vi "Sondenmodell.Erdtemperatur.vi"(8 "Error in":errorcluster, 10 "Vorlauftemperatur Solekreislauf [°C]":dbl, 11 "Sondenmodell in":refnum<data-value>) -> (0 "Error out":errorcluster, 3 "Sondenmodell out":refnum<data-value>)   [LabVIEW 2016, in "Sondenmodell.lvclass"]
uses:
  Sondenmodell.lvclass
  Sondenmodell.lvclass/Sondenmodell.ctl
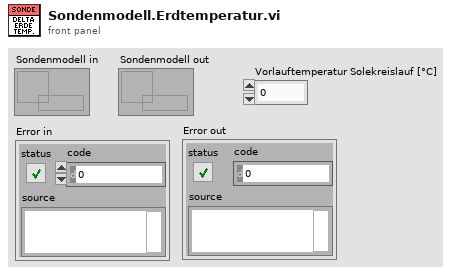
[diagram p1: front panel]
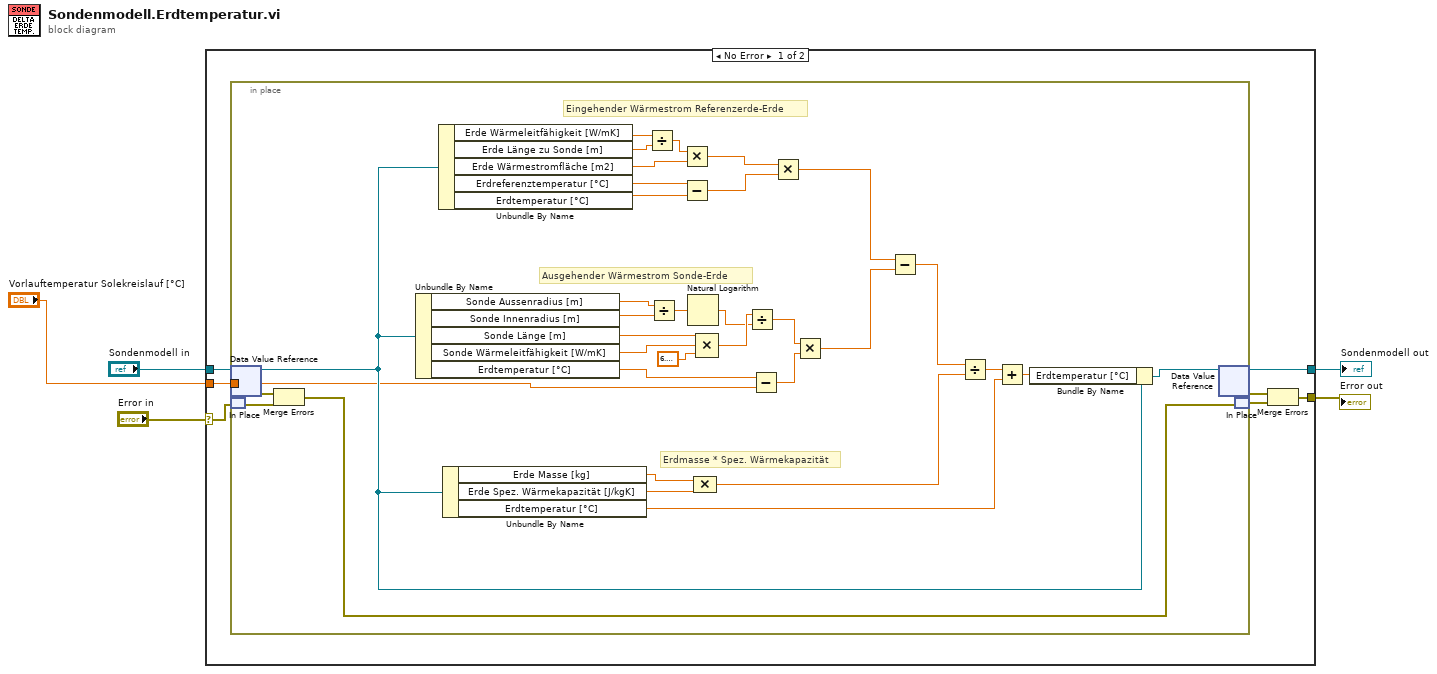
[diagram p0: block diagram]
diagram:
  n1 = case shown="No Error" "Error in" {
    selector: "Error in" -> [w9 w47]
    tunnel: "Sondenmodell in" -> [w10 w48]
    tunnel: [w8 w48] -> w3
    tunnel: [w7 w47] -> w2
    tunnel: "Vorlauftemperatur Solekreislauf [°C]" -> [w6 _]
    frame No Error {
      n2 = in-place {
        in-place-border: w6 -> [w13]
        # "Erdmasse * Spez. Wärmekapazität"
        # "Ausgehender Wärmestrom Sonde-Erde"
        # "Eingehender Wärmestrom Referenzerde-Erde"
        n3 = in-place-dvr #1(w10) -> (w16:refnum<class "Sondenmodell.lvclass">, w46:errorcluster)
        n4 = in-place-match #2(w9) -> (w45:errorcluster)
        n5 = Merge Errors(w46, w45) -> (w15:errorcluster)
        n6 = Unbundle By Name(w16) -> ("Sonde Aussenradius [m]"=w29:dbl, "Sonde Innenradius [m]"=w28:dbl, "Sonde Länge [m]"=w26:dbl, "Sonde Wärmeleitfähigkeit [W/mK]"=w25:dbl, "Erdtemperatur [°C]"=w23:dbl)
        n7 = Unbundle By Name(w16) -> ("Erde Wärmeleitfähigkeit [W/mK]"=w34:dbl, "Erde Länge zu Sonde [m]"=w33:dbl, "Erde Wärmestromfläche [m2]"=w31:dbl, "Erdreferenztemperatur [°C]"=w30:dbl, "Erdtemperatur [°C]"=w39:dbl)
        n8 = Unbundle By Name(w16) -> ("Erde Masse [kg]"=w36:dbl, "Erde Spez. Wärmekapazität [J/kgK]"=w14:dbl, "Erdtemperatur [°C]"=w37:dbl)
        n9 = Divide(x=w34, y=w33) -> (x/y=w32:dbl)
        n10 = Divide(x=w29, y=w28) -> (x/y=w27:dbl)
        n11 = Multiply(x=w32, y=w31) -> (x*y=w44:dbl)
        n12 = Subtract(x=w30, y=w39) -> (x-y=w43:dbl)
        n13 = Natural Logarithm(1:w27) -> (0:w21:dbl)
        n14 = Compound Arithmetic op=MULTIPLY(w36, w14) -> (w35:dbl)
        n15 = Compound Arithmetic op=MULTIPLY(w26, w25, 6.283185307179586) -> (w22:dbl)
        n16 = Divide(x=w22, y=w21) -> (x/y=w20:dbl)
        n17 = Subtract(x=w23, y=w13) -> (x-y=w19:dbl)
        n18 = Multiply(x=w44, y=w43) -> (x*y=w42:dbl)
        n19 = Multiply(x=w20, y=w19) -> (x*y=w18:dbl)
        n20 = Subtract(x=w42, y=w18) -> (x-y=w41:dbl)
        n21 = Divide(x=w41, y=w35) -> (x/y=w40:dbl)
        n22 = Add(x=w40, y=w37) -> (x+y=w38:dbl)
        n23 = Bundle By Name(cluster=w16, "Erdtemperatur [°C]"=w38) -> (w17:refnum<class "Sondenmodell.lvclass">)
        n24 = in-place-dvr #1(w17) -> (w8:refnum<data-value>, w12:errorcluster)
        n25 = in-place-match #2(w15) -> (w11:errorcluster)
      }
      n26 = Merge Errors(w12, w11) -> (w7:errorcluster)
    }
    frame Error {
    }
  }
  "Sondenmodell out" <- w3
  "Error out" <- w2
